vi "Core-Engine.vi"(7 "Ctrl-Refs":T1, 8 "Err-I":errorcluster, 9 "ErrQRef":refnum<queue>, 11 "MainQ-I":refnum<queue>) -> (0 "Err-O":errorcluster)   [LabVIEW 2020]
doc: "Main State Machine LOOP of Core.\nThis vi act as an engine to pump application run."
uses:
  Core-CtrlRefs.ctl
panel:
  # "Outputs"
  # "Inputs"
  # ":: Modularized Parallism Templete ::\n- Main State Machine -\nby: Techie <HighTechYoung@yahoo.com>\nhttp://www.Vigo-tech.com\nCopyright (C) 2010, Vigo Technologies All Rights Reserved"
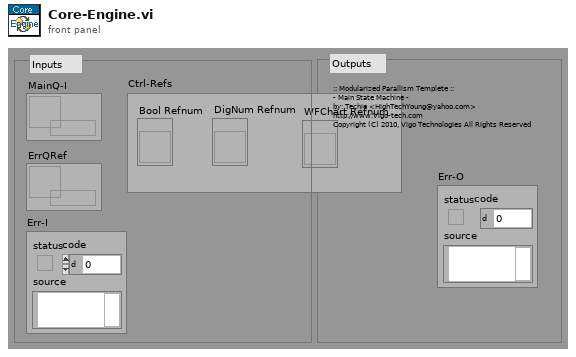
[diagram p1: front panel]
types:
  T1 = typedef "Core-CtrlRefs.ctl" = cluster{"Bool Refnum":refnum<vi>, "DigNum Refnum":refnum<vi>, "WFChart Refnum":refnum<vi>}
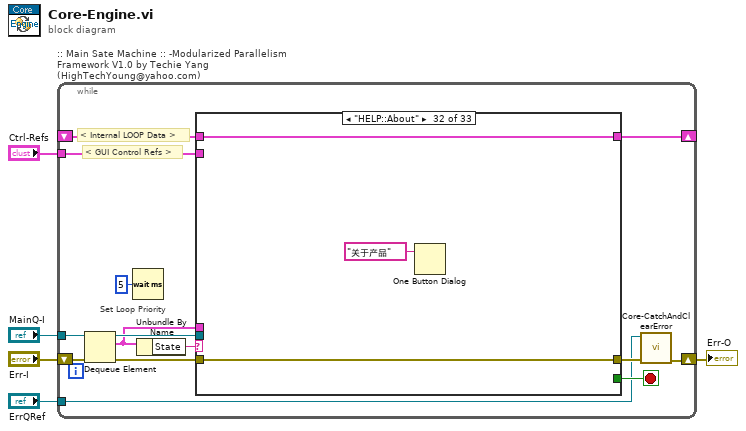
[diagram p0: block diagram]
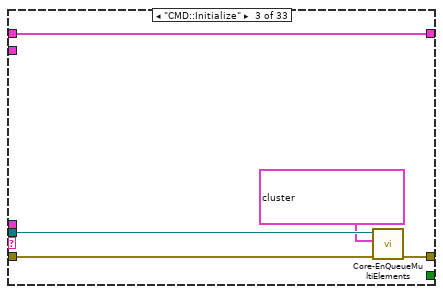
[diagram p4: hidden frame]
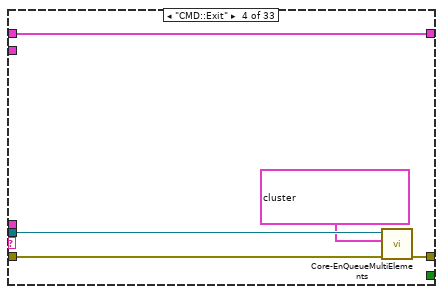
[diagram p5: hidden frame]
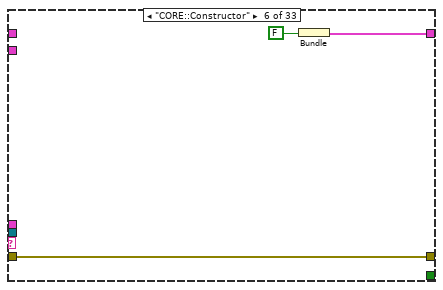
[diagram p7: hidden frame]
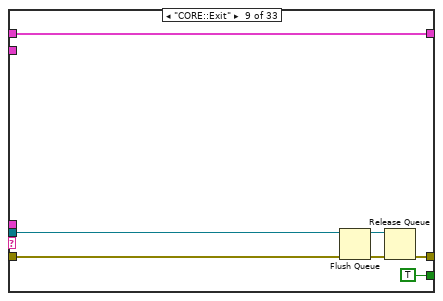
[diagram p10: hidden frame]
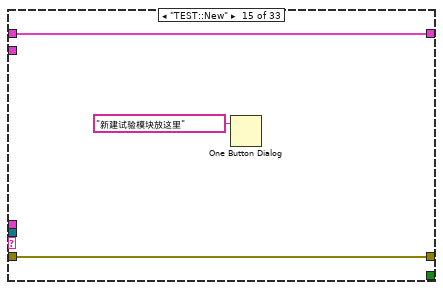
[diagram p16: hidden frame]
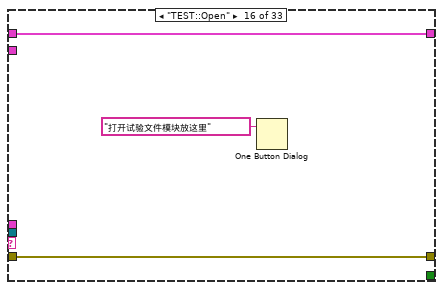
[diagram p17: hidden frame]
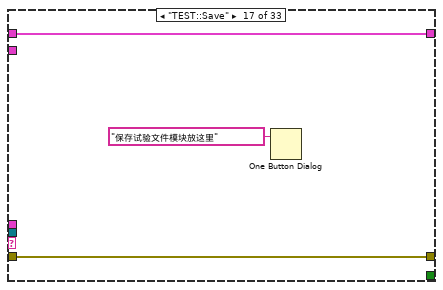
[diagram p18: hidden frame]
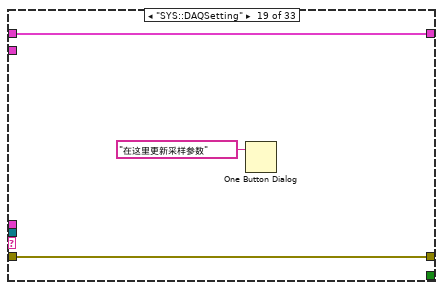
[diagram p20: hidden frame]
diagram:
  n1 = while ":: Main Sate Machine :: -Modularized Parallelism Framework V1.0 by Techie Yang (HighTechYoung@yahoo.com)" {
    tunnel: "MainQ-I" -> [w19]
    shift-right: [w8] -> w2
    shift-left: "Err-I" -> [w10]
    shift-right: [w13] -> _
    shift-left: _ -> [w12]
    tunnel: "Ctrl-Refs" -> [w11]
    tunnel: "ErrQRef" -> [w7]
    stop <- w16 stop-if-true
    # "Set Loop Priority"
    # "< GUI Control Refs >"
    # "< Internal LOOP Data >"
    n2 = Dequeue Element(queue=w19, error in (no error)=w10) -> (queue out=w17:refnum<queue>, element=w14:cluster{"State":string, "Data":variant}, error out=w18:errorcluster)  [unwired: 2 out]
    n3 = Wait (ms)(milliseconds to wait=u32 5) -> ()  [unwired: 1 out]
    n4 = Unbundle By Name(w14) -> ("State"=w15:string)
    n5 = case shown="\"HELP::About\"" w15 {
      tunnel: [w20 w23 w27 w32 w35 w38 w40 w42 w45 w50 w52 w54 w57 w59 w62 w64 w68 w70 w73 w75 w78 w82 w85 w88 w90 w93 w95 w99 w102 w105 w106 w109 w113] -> w9
      tunnel: [_ _ _ _ _ _ _ _ TRUE _ _ _ _ _ _ _ _ _ _ _ _ _ _ _ _ _ _ _ _ _ _ _ _] -> w16
      tunnel: w17 -> [_ _ w28 w31 _ _ _ _ w48 _ _ _ _ _ _ _ _ _ _ _ _ _ _ _ _ _ _ _ _ _ _ _ _]
      tunnel: w18 -> [w20 w23 w24 w33 w35 w38 w40 w42 w47 w50 w52 w54 w57 w59 w62 w64 w68 w70 w73 w75 w78 w82 w85 w88 w90 w93 w95 w99 w102 w105 w106 w109 w113]
      tunnel: w14 -> [_ _ _ _ _ _ _ _ _ _ _ _ _ _ _ _ _ _ _ _ _ _ _ _ _ _ _ _ _ _ _ _ _]
      tunnel: [w21 w22 w25 w29 w34 w36 w39 w41 w43 w51 w53 w55 w56 w58 w60 w63 w67 w69 w72 w74 w79 w80 w84 w87 w89 w92 w96 w98 w101 w104 w107 w110 w112] -> w13
      tunnel: w12 -> [w21 w22 w25 w29 w34 _ w39 w41 w43 w51 w53 w55 w56 w58 w60 w63 w67 w69 w72 w74 w79 w80 w84 w87 w89 w92 w96 w98 w101 w104 w107 w110 w112]
      tunnel: w11 -> [_ _ _ _ _ _ _ _ _ _ _ _ _ _ _ _ _ _ _ _ _ _ _ _ _ _ _ _ _ _ _ _ _]
      frame "IDLE", Default {
      }
      frame "-------- Commands ---------" {
      }
      frame "CMD::Initialize" {
        n6 = call "Core-EnQueueMultiElements.vi"("ErrorIn"=w24, "CmdArray"=cluster{"State":string, "Data":variant}[] [{"State"="CORE::Constructor", "Data"=variant}, {"State"="CORE::Initialize", "Data"=variant}], "QRefIn"=w28) -> ("ErrorOut"=w27:errorcluster)  [unwired: 8 in]
      }
      frame "CMD::Exit" {
        n7 = call "Core-EnQueueMultiElements.vi"("ErrorIn"=w33, "CmdArray"=cluster{"State":string, "Data":variant}[] [{"State"="CORE::DeConstructor", "Data"=variant}, {"State"="CORE::Exit", "Data"=variant}], "QRefIn"=w31) -> ("ErrorOut"=w32:errorcluster)  [unwired: 8 in]
      }
      frame "------------ Core ------------" {
      }
      frame "CORE::Constructor" {
        n8 = Bundle(FALSE) -> (w36:cluster{bool})  [unwired: 1 in]
      }
      frame "CORE::Initialize" {
      }
      frame "CORE::DeConstructor" {
      }
      frame "CORE::Exit" {
        n9 = Flush Queue(queue=w48, error in (no error)=w47) -> (queue out=w44:refnum<queue>, error out=w46:errorcluster)  [unwired: 1 out]
        n10 = Release Queue(queue=w44, error in (no error)=w46) -> (error out=w45:errorcluster)  [unwired: 1 in, 2 out]
      }
      frame "------------  GUI  -------------" {
      }
      frame "GUI::Initialize" {
      }
      frame "GUI::SetCusor" {
      }
      frame "GUI::SetMenu" {
      }
      frame "------------  TEST -------------" {
      }
      frame "TEST::New" {
        n11 = One Button Dialog(message="新建试验模块放这里") -> ()  [unwired: 1 in, 1 out]
      }
      frame "TEST::Open" {
        n12 = One Button Dialog(message="打开试验文件模块放这里") -> ()  [unwired: 1 in, 1 out]
      }
      frame "TEST::Save" {
        n13 = One Button Dialog(message="保存试验文件模块放这里") -> ()  [unwired: 1 in, 1 out]
      }
      frame "------------  PARAM -------------" {
      }
      frame "SYS::DAQSetting" {
        n14 = One Button Dialog(message="在这里更新采样参数") -> ()  [unwired: 1 in, 1 out]
      }
      frame "SYS::CurveParam" {
        n15 = One Button Dialog(message="ÔÚÕâÀïÅäÖÃÇúÏß²ÎÊý£") -> ()  [unwired: 1 in, 1 out]
      }
      frame "SYS::Config" {
        n16 = One Button Dialog(message="在这里配置系统参数") -> ()  [unwired: 1 in, 1 out]
      }
      frame "SYS::Serial" {
        n17 = One Button Dialog(message="串口配置") -> ()  [unwired: 1 in, 1 out]
      }
      frame "SYS::Sensor1" {
        n18 = One Button Dialog(message="#1扭矩传感器参数") -> ()  [unwired: 1 in, 1 out]
      }
      frame "SYS::Sensor2" {
        n19 = One Button Dialog(message="#2扭矩传感器参数") -> ()  [unwired: 1 in, 1 out]
      }
      frame "-------CURVE-REPORT -----------" {
      }
      frame "CURVE::AL" {
        n20 = One Button Dialog(message="曲线分析") -> ()  [unwired: 1 in, 1 out]
      }
      frame "RPT::Set" {
        n21 = One Button Dialog(message="报表设置") -> ()  [unwired: 1 in, 1 out]
      }
      frame "RPT::Go" {
        n22 = One Button Dialog(message="试验报告") -> ()  [unwired: 1 in, 1 out]
      }
      frame "DATA::Expt" {
        n23 = One Button Dialog(message="数据导出") -> ()  [unwired: 1 in, 1 out]
      }
      frame "DATA::BlkBox" {
        n24 = One Button Dialog(message="查看黑盒子数据") -> ()  [unwired: 1 in, 1 out]
      }
      frame "------- HELP -----------" {
      }
      frame "HELP::About" {
        n25 = One Button Dialog(message="关于产品") -> ()  [unwired: 1 in, 1 out]
      }
      frame "HELP::Service" {
        n26 = One Button Dialog(message="售后服务") -> ()  [unwired: 1 in, 1 out]
      }
    }
    n27 = call "Core-CatchAndClearError.vi"("Err-I"=w9, "ErrQ-I"=w7) -> ("Err-O"=w8:errorcluster)  [unwired: 9 in]
  }
  "Err-O" <- w2
